vi "菜单-导出py.vi"(8 "error in (no error)":errorcluster caption="错误输入（无错误）", 11 "程序响应 输入":refnum<class "程序响应.lvclass">) -> (0 "error out":errorcluster caption="错误输出", 3 "程序响应 输出":refnum<class "程序响应.lvclass">)   [LabVIEW 2020, in "程序响应.lvlib" / "程序响应.lvclass"]
uses:
  D:/SuperPython-master/ScintillaNET.dll
  ScintillaNET.dll
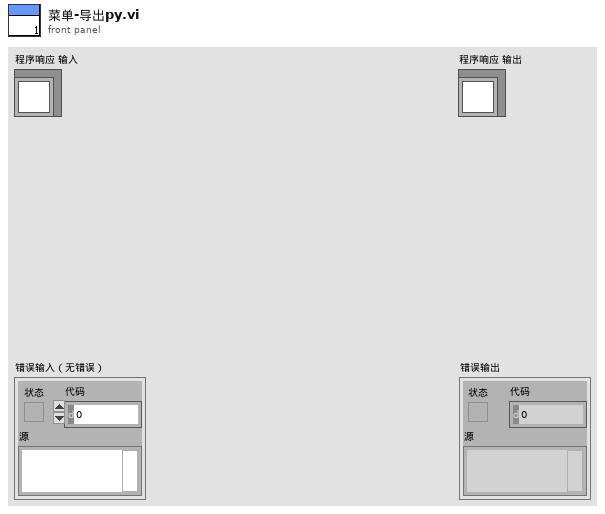
[diagram p1: front panel]
types:
  T1 = enum16{"open", "replace", "create", "open or create", "replace or create", "replace or create with confirmation"}
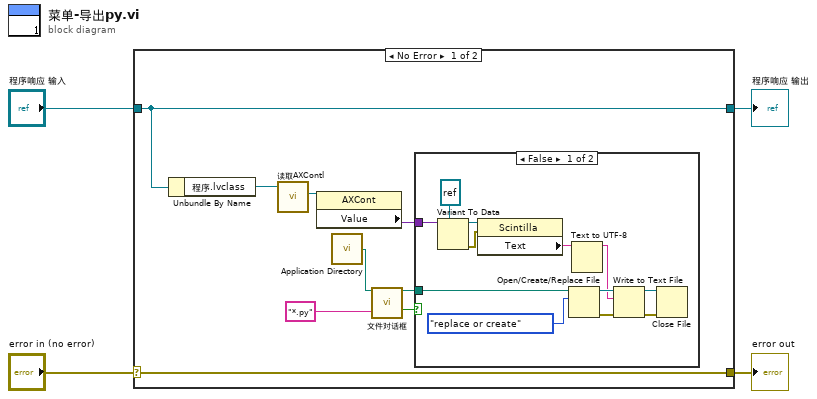
[diagram p0: block diagram]
diagram:
  n1 = case shown="No Error" "error in (no error)" {
    selector: "error in (no error)" -> [w13 w27]
    tunnel: [w13 w27] -> w3
    tunnel: [w12 w26] -> w1
    tunnel: "程序响应 输入" -> [w12 w26]
    frame No Error {
      n2 = Unbundle By Name(w12) -> ("程序.lvclass"=w6:refnum<class "程序.lvclass">)
      n3 = call-dynamic "读取AXContl.vi"("程序输入"=w6) -> ("AXContl"=w5:refnum<vi>)  [unwired: 8 in, 2 out]
      n4 = property class="AXCont"(reference=w5) -> ("Value"=w9:variant)  [unwired: 1 in, 2 out]
      n5 = call <vilib>:"Application Directory.vi"() -> ("Application Directory"=w10:path)
      n6 = call "文件对话框"("start path"=w10, "pattern (all files)"="*.py") -> ("selected path"=w11:path, "cancelled"=w7:bool)  [unwired: 10 in, 2 out]
      n7 = case shown="False" w7 {
        tunnel: w11 -> [w20 _]
        tunnel: w9 -> [w16 _]
        frame False {
          n8 = Variant To Data(type=refnum<k24> refnum ("文本编辑"), Variant=w16) -> (data=w17:refnum<k24>, error out=w18:errorcluster)  [unwired: 1 in]
          n9 = property class="Scintilla"(reference=w17, error in=w18) -> ("Text"=w15:string)  [unwired: 2 out]
          n10 = Open/Create/Replace File(file path (use dialog)=w20, operation (0:open)=T1."replace or create" ("操作(0:open)")) -> (refnum out=w25:refnum<file>, error out=w24:errorcluster)  [unwired: 4 in, 1 out]
          n11 = Text to UTF-8 ("文本至UTF-8转换")(11:w15) -> (3:w14:string)  [unwired: 2 in, 1 out]
          n12 = Write to Text File(file (use dialog)=w25, text=w14, error in=w24) -> (refnum out=w23:refnum<file>, error out=w22:errorcluster)  [unwired: 1 in, 1 out]
          n13 = Close File(refnum=w23, error in=w22) -> ()  [unwired: 2 out]
        }
        frame True {
        }
      }
    }
    frame Error {
    }
  }
  "error out" <- w3
  "程序响应 输出" <- w1
